vi "LVSWrt_Rd.vi"(9 "WriteBuf":string="?", 11 "COM Port":refnum<visa-resource-name>) -> (0 "error out":errorcluster, 2 "string read":string)   [LabVIEW 2017]
uses:
  instr.lib/lvserial/lvserial.lvlib
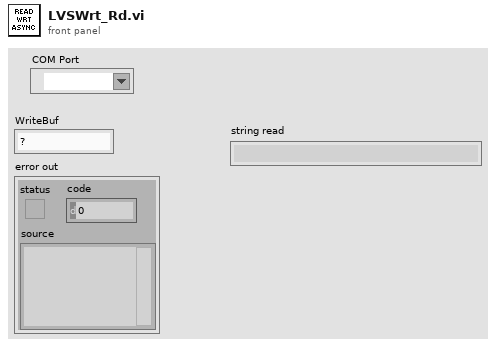
[diagram p1: front panel]
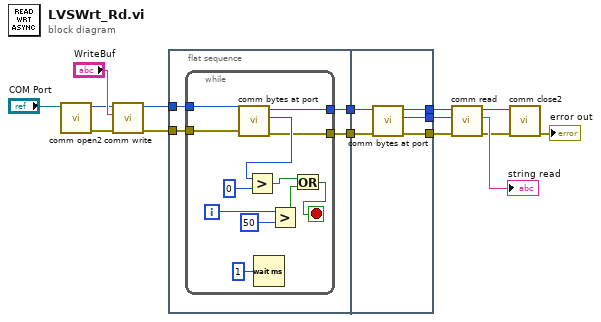
[diagram p0: block diagram]
diagram:
  n1 = call "comm open2.vi"("Comm Port Name"="COM Port") -> ("error out"=w1:errorcluster, "Comm Handle"=w2:u32)  [unwired: 4 in, 1 out]
  n2 = call "comm write.vi"("error in (no error)"=w1, "string to write"="WriteBuf", "Comm Handle"=w2) -> ("error out"=w3:errorcluster, "dup Comm Handle"=w4:u32)  [unwired: 6 in, 1 out]
  n3 = flat-sequence {
    tunnel: w4 -> [w19]
    tunnel: w3 -> [w18]
    tunnel: [w17] -> w10
    tunnel: [w16] -> w9
    tunnel: [w36] -> w11
    tunnel: w10 -> [w35]
    tunnel: w9 -> [w34]
    tunnel: [w33] -> w6
    tunnel: [w32] -> w5
    frame #0 {
      n4 = while {
        tunnel: w19 -> [w23]
        tunnel: w18 -> [w22]
        tunnel: [w21] -> w17
        tunnel: [w20] -> w16
        i -> [w24]
        stop <- w26 stop-if-true
        n5 = call "comm bytes at port.vi"("error in (no error)"=w22, "Comm Handle"=w23) -> ("error out"=w20:errorcluster, "bytes at port"=w25:u32, "dup Comm Handle"=w21:u32)  [unwired: 7 in]
        n6 = Greater?(x=w25, y=u32 0) -> (0:w29:bool)
        n7 = Wait (ms)(milliseconds to wait=u32 1) -> ()  [unwired: 1 out]
        n8 = Greater?(x=w24, y=50) -> (0:w30:bool)
        n9 = Or(x=w29, y=w30) -> (x .or. y?=w26:bool)
      }
    }
    frame #1 {
      n10 = call "comm bytes at port.vi"("error in (no error)"=w34, "Comm Handle"=w35) -> ("error out"=w32:errorcluster, "bytes at port"=w36:u32, "dup Comm Handle"=w33:u32)  [unwired: 7 in]
    }
  }
  n11 = call "comm read.vi"("error in (no error)"=w5, "requested byte count"=w11, "Comm Handle"=w6) -> ("error out"=w7:errorcluster, "string read"=→"string read":string, "dup Comm Handle"=w14:u32)  [unwired: 5 in, 1 out]
  n12 = call "comm close2.vi"("error in (no error)"=w7, "Comm Handle"=w14) -> ("error out"=→"error out":errorcluster)  [unwired: 5 in]
